vi "Get Status.vi"(8 "error in (no error)":errorcluster, 11 "bt_System in":refnum<class "bt_System.lvclass">) -> (0 "error out":errorcluster, 2 "Status":T1, 3 "bt_System out":refnum<class "bt_System.lvclass">)   [LabVIEW 2021, in "BT.lvlib" / "bt_System.lvclass"]
uses:
  bt_System.lvclass
  bt_System.lvclass/bt_System.ctl
  Support/Nodes/abs_Node/Status.ctl
  Support/Nodes/abs_Node/bt_Node.lvclass
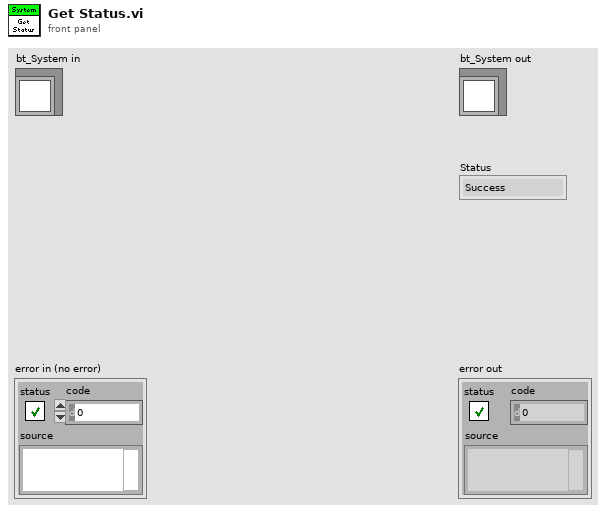
[diagram p1: front panel]
types:
  T1 = typedef "BT.lvlib/bt_Node.lvclass/Status.ctl" = enum16{"Success", "Failure", "Running"}
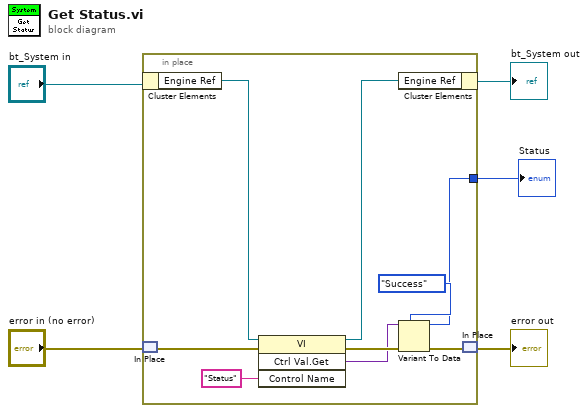
[diagram p0: block diagram]
diagram:
  n1 = in-place {
    in-place-border: [w8] -> w3
    n2 = in-place-cluster #1("bt_System in") -> ("Engine Ref"=w14:refnum<vi>)
    n3 = in-place-match #2("error in (no error)") -> (w7:errorcluster)
    n4 = invoke class="VI" method="Ctrl Val.Get"(reference=w14, error in=w7, "Control Name"="Status") -> (reference out=w13:refnum<vi>, error out=w11:errorcluster, "Get Control Value Variant"=w10:variant)  [unwired: 1 in, 1 out]
    n5 = in-place-cluster #1("Engine Ref"=w13) -> (→"bt_System out":refnum<class "bt_System.lvclass">)
    n6 = Variant To Data(error in=w11, type=Status."Success" ("Status"), Variant=w10) -> (data=w8:T1, error out=w6:errorcluster)
    n7 = in-place-match #2(w6) -> (→"error out":errorcluster)
  }
  "Status" <- w3
